vi "7260 Read.vi"(8 "error in (no error)":errorcluster, 11 "VISA Resource Name":refnum<visa-resource-name>) -> (0 "error out":errorcluster, 1 "Y":dbl format="%.4e", 2 "X":dbl format="%.4e", 3 "VISA Resource Name Out":refnum<visa-resource-name>, 4 "data string":string)   [LabVIEW 2021]
uses:
  GPIB/VISA  Send Receive.vi
  Simple VISA Reader/Simple VISA Reader Driver.lvclass
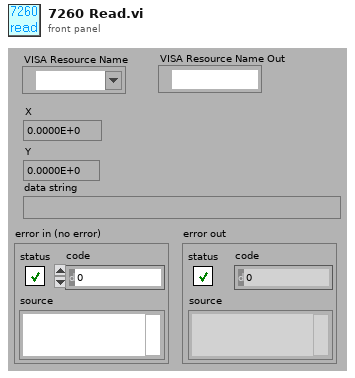
[diagram p1: front panel]
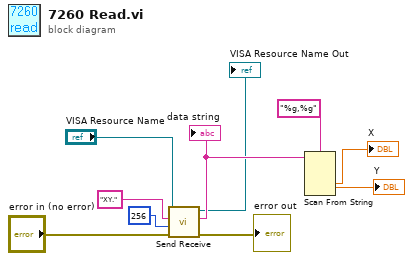
[diagram p0: block diagram]
diagram:
  n1 = call-poly "Send Receive.vi"("error in (no error)"="error in (no error)", "Receive count"=256 ("count"), "data string in"="XY." ("data string"), "VISA Resource Name"="VISA Resource Name") -> ("error out"=→"error out":errorcluster, "data string out"=w5:string, "VISA Resource Name Out"=→"VISA Resource Name Out":refnum<visa-resource-name>)  [unwired: 5 in]
  "data string" <- w5
  n2 = Scan From String(format string="%g,%g", input string=w5) -> (output 1=→"X":dbl, output 2=→"Y":dbl)  [unwired: 2 in, 5 out]
